vi "HovaCAL_Interface_SetPumpParameter.vi"(8 "error in (no error)":errorcluster caption="Fehler (Eingang, kein Fehler)", 10 "Pump Idx":i32, 11 "Komponent Name":string) -> (0 "error out":errorcluster caption="Fehler (Ausgang)")   [LabVIEW 2020, in "Linearisierung v2.lvlib" / "Gasteiler.lvlib" / "HovaCAL_Interface.lvlib" / "Kommunikation.lvlib"]
uses:
  Kommunikation.lvlib
  Aktion_FGV_HovaCAL_Interface_SetData.ctl
  Controls/Pump Concentration Mode.ctl
  Aktion_FGV_HovaCAL_Interface_Kommunikation.ctl
  Aktion_FGV_HovaCAL_Interface_Kommandos.ctl
  Controls/Controls.lvlib
  Controls/Pump Control Mode.ctl
  Controls/Pump Dry Mode.ctl
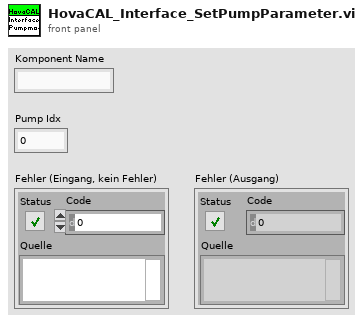
[diagram p1: front panel]
types:
  T1 = typedef "Linearisierung v2.lvlib/Gasteiler.lvlib/HovaCAL_Interface.lvlib/Controls.lvlib/Pump Dry Mode.ctl" = i32
  T2 = typedef "Linearisierung v2.lvlib/Gasteiler.lvlib/HovaCAL_Interface.lvlib/Controls.lvlib/Pump Control Mode.ctl" = u32
  T3 = typedef "Linearisierung v2.lvlib/Gasteiler.lvlib/HovaCAL_Interface.lvlib/Controls.lvlib/Pump Concentration Mode.ctl" = i32
  T4 = typedef "Linearisierung v2.lvlib/Gasteiler.lvlib/HovaCAL_Interface.lvlib/Kommunikation.lvlib/Aktion_FGV_HovaCAL_Interface_SetData.ctl" = enum16{"lesen", "Konzentrationen", "Pumpen Parameter", "Pumpe Konzentration", "Pumpe run", "Temperaturen", "Fluss", "Limits", "init"}
  T5 = cluster{"running?":bool, "dry mode":T1, "control mode":T2}
  T6 = typedef "Linearisierung v2.lvlib/Gasteiler.lvlib/HovaCAL_Interface.lvlib/Controls.lvlib/Reagent.ctl" = i32
  T7 = cluster{"concentratio mode":T3, "Reagent":T6, "Molarity":dbl, "density":dbl, "syringe":dbl, "pump_a":dbl}[]
  T8 = cluster{"concentratio mode":T3, "Reagent":T6, "Molarity":dbl, "density":dbl, "syringe":dbl, "pump_a":dbl}
  T9 = typedef "Linearisierung v2.lvlib/Gasteiler.lvlib/HovaCAL_Interface.lvlib/Kommunikation.lvlib/Aktion_FGV_HovaCAL_Interface_Kommandos.ctl" = enum16{"lesen", "verarbeiten", "hinzufügen", "on top", "init", "sammeln", "freigeben", "connected"}
  T10 = typedef "Linearisierung v2.lvlib/Gasteiler.lvlib/HovaCAL_Interface.lvlib/Kommunikation.lvlib/Aktion_FGV_HovaCAL_Interface_Kommunikation.ctl" = enum16{"Initialisieren", "Set Konzentrationen", "Set Gase", "Set Limits", "Get Dynamische Werte", "Beenden", "Com ändern", "Get Gase init", "Pause", "Get Gasteiler Infos", "Get MFC Infos", "Set Pumpen Parameter", "Set Pumpe Konzenration", "Set Pumpe run", "Set Temperaturen", "Set Fluss", "Get Gase", "Get Limits", "Get Dynamische Werte 1", "Get Dynamische Werte 2"}
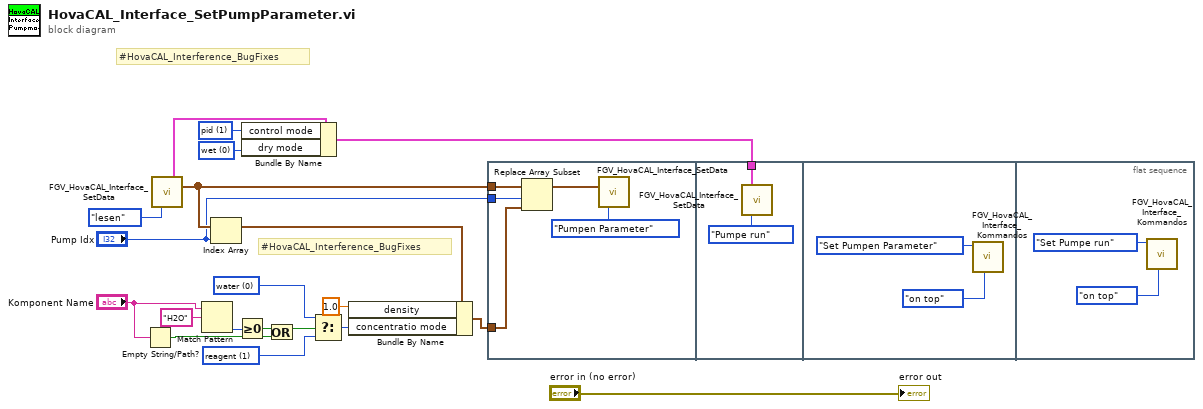
[diagram p0: block diagram]
diagram:
  w1 = T1 0 items=["wet", "dry"] ("dry mode")
  w3 = T2 1 items=["static", "pid"] ("control mode")
  w10 = T3 1 items=["water", "reagent"] ("concentratio mode")
  w11 = T3 0 items=["water", "reagent"] ("concentratio mode")
  # "#HovaCAL_Interference_BugFixes"
  # "#HovaCAL_Interference_BugFixes"
  n1 = Empty String/Path?(string/path="Komponent Name") -> (empty?=w6:bool)
  n2 = call "FGV_HovaCAL_Interface_SetData.vi"("Aktion"=Aktion_FGV_HovaCAL_Interface_SetData."lesen") -> ("PumpModeGeneral-Cluster out"=w4:T5, "PumpMode-Cluster out"=w15:T7)  [unwired: 8 in, 5 out]
  n3 = Match Pattern(string="Komponent Name", regular expression="H2O" ("Regulärer Ausdruck")) -> (offset past match=w13:i32)  [unwired: 1 in, 3 out]
  n4 = Index Array(array=w15, index="Pump Idx") -> (element=w16:T8)
  n5 = Greater Or Equal To 0?(x=w13) -> (x >= 0?=w12:bool)
  n6 = Bundle By Name(cluster=w4, "control mode"=w3, "dry mode"=w1) -> (w2:T5)
  n7 = Or(x=w12, y=w6) -> (x .or. y?=w7:bool)
  n8 = Select(t=w11, s=w7, f=w10) -> (s? t:f=w9:T3)
  n9 = Bundle By Name(cluster=w16, "density"=1.0, "concentratio mode"=w9) -> (w20:T8)
  n10 = flat-sequence {
    tunnel: w20 -> [w22]
    tunnel: w15 -> [w24]
    tunnel: "Pump Idx" -> [w23]
    tunnel: w2 -> [w26]
    frame #0 {
      n11 = Replace Array Subset(array=w24, new element=w22, index=w23) -> (w21:T7)
      n12 = call "FGV_HovaCAL_Interface_SetData.vi"("PumpMode-Cluster in"=w21, "Aktion"=Aktion_FGV_HovaCAL_Interface_SetData."Pumpen Parameter") -> ()  [unwired: 7 in, 7 out]
    }
    frame #1 {
      n13 = call "FGV_HovaCAL_Interface_SetData.vi"("PumpModeGeneral-Cluster in"=w26, "Aktion"=Aktion_FGV_HovaCAL_Interface_SetData."Pumpe run") -> ()  [unwired: 7 in, 7 out]
    }
    frame #2 {
      n14 = call "FGV_HovaCAL_Interface_Kommandos.vi"("Aktion"=Aktion_FGV_HovaCAL_Interface_Kommandos."on top", "Kommando in"=Aktion_FGV_HovaCAL_Interface_Kommunikation."Set Pumpen Parameter") -> ()  [unwired: 3 in, 6 out]
    }
    frame #3 {
      n15 = call "FGV_HovaCAL_Interface_Kommandos.vi"("Aktion"=Aktion_FGV_HovaCAL_Interface_Kommandos."on top", "Kommando in"=Aktion_FGV_HovaCAL_Interface_Kommunikation."Set Pumpe run") -> ()  [unwired: 3 in, 6 out]
    }
  }
  "error out" <- "error in (no error)"
